vi "CenterCrosshair.vi"(4 "Y Resolution":i32, 6 "X Resolution":i32, 11 "Image In":T1) -> (3 "Image Out":T1)   [LabVIEW 2012]
uses:
  <vilib>/vision/Image Controls.llb/IMAQ Image.ctl
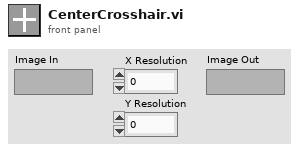
[diagram p1: front panel]
types:
  T1 = typedef "IMAQ Image.ctl" = refnum<image>
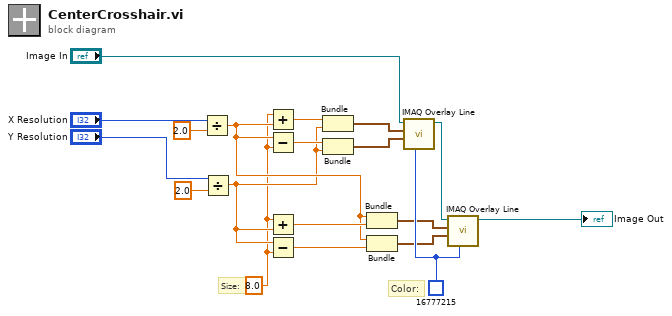
[diagram p0: block diagram]
diagram:
  w19 = u32 16777215 ("Color")
  w3 = 8.0 ("x")
  # "Color:"
  # "Size:"
  n1 = Divide(x="X Resolution", y=2.0) -> (x/y=w7:dbl)
  n2 = Divide(x="Y Resolution", y=2.0) -> (x/y=w6:dbl)
  n3 = Add(x=w3, y=w7) -> (x+y=w17:dbl)
  n4 = Subtract(x=w7, y=w3) -> (x-y=w18:dbl)
  n5 = Add(x=w3, y=w6) -> (x+y=w12:dbl)
  n6 = Subtract(x=w6, y=w3) -> (x-y=w11:dbl)
  n7 = Bundle(w17, w6) -> (w16:cluster{dbl, dbl})  [unwired: 1 in]
  n8 = Bundle(w18, w6) -> (w15:cluster{dbl, dbl})  [unwired: 1 in]
  n9 = Bundle(w7, w12) -> (w14:cluster{dbl, dbl})  [unwired: 1 in]
  n10 = Bundle(w7, w11) -> (w13:cluster{dbl, dbl})  [unwired: 1 in]
  n11 = call "IMAQ Overlay Line"("Color"=w19, "End Point"=w15, "Start Point"=w16, "Image"="Image In") -> ("Image Out"=w10:T1)  [unwired: 6 in, 1 out]
  n12 = call "IMAQ Overlay Line"("Color"=w19, "End Point"=w13, "Start Point"=w14, "Image"=w10) -> ("Image Out"=→"Image Out":T1)  [unwired: 6 in, 1 out]
